vi "Clear Task.vi"(8 "error in":errorcluster, 11 "NI Digital Output in":refnum<class "NI Digital Output.lvclass">) -> (0 "error out":errorcluster, 3 "NI Digital Output out":refnum<class "NI Digital Output.lvclass">)   [LabVIEW 2023, in "HardwareAbstractionLayer_LVOOP.lvlib" / "NI Digital Output.lvclass"]
doc: "DAQ AO Clear Data"
uses:
  NI Digital Output.lvclass
  NI Digital Output.lvclass/NI Digital Output.ctl
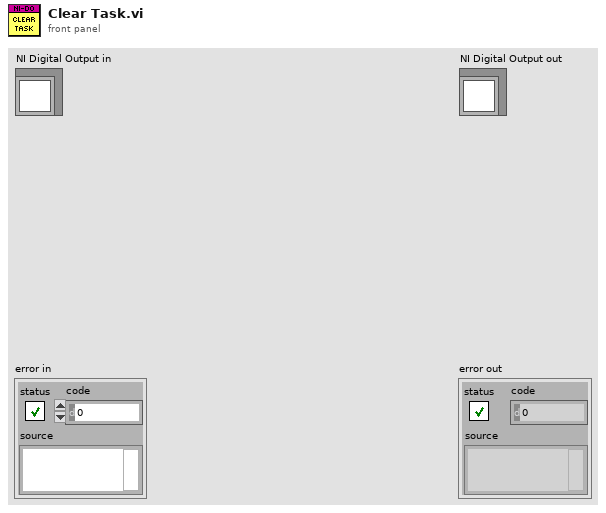
[diagram p1: front panel]
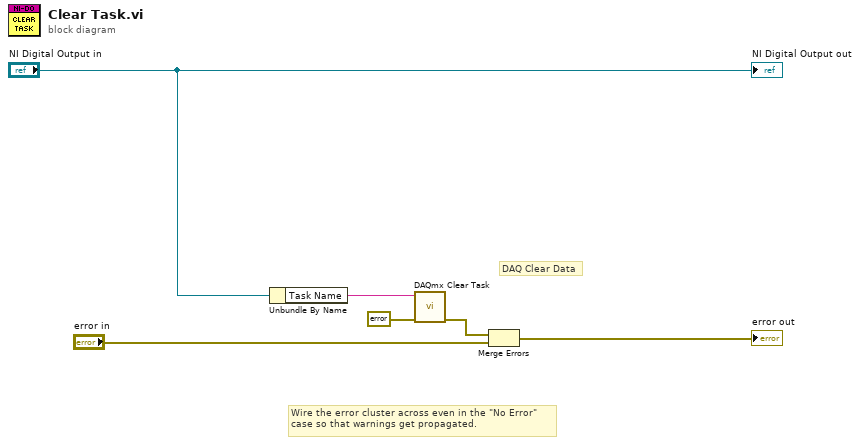
[diagram p0: block diagram]
diagram:
  # "DAQ Clear Data"
  # "Wire the error cluster across even in the \"No Error\"\ncase so that warnings get propagated."
  n1 = Unbundle By Name("NI Digital Output in") -> ("Task Name"=w2:string)
  n2 = call <vilib>:"DAQmx Clear Task.vi"("task in"=w2, "error in"=errorcluster {"status"=FALSE, "code"=0, "source"=""}) -> ("error out"=w3:errorcluster)  [unwired: 13 in]
  n3 = Merge Errors(w3, "error in") -> (→"error out":errorcluster)
  "NI Digital Output out" <- "NI Digital Output in"
